vi "Main.vi"() -> ()   [LabVIEW 2013]
doc: "This is the main VI and the GUI for configuring and using the AFM."
uses:
  subvi/simulator/Global Variables.vi
panel:
  out "Function generator waveform display":cluster{dbl[], "Y":dbl[]}(graph)
  out "Sample Size":cluster{"Width (µm)":dbl, "Height (µm)":dbl}={"Width (µm)"=40.0, "Height (µm)"=40.0}
  in  "update X/Y?":bool
  in  "Open simulator?":bool
  out "Rendered Image":T1(plugin-control)
  in  "Settings":T2(tab)=enum."Inkscape Design and Background Image"
  in  "Function generator":T3(array[cluster])=[{"Max Voltage"=10.0, "Min Voltage"=-2.0, "signal type"=enum."Square Wave", "square wave duty cycle (%)"=90.0, "Cycle number"=100.0, "Phase"=0.0}] {"square wave duty cycle (%)" format="%0.2f"}
  in  "Same setting":bool=TRUE
  in  "Same setting":bool=TRUE
  in  "Rectangle Properties":T4(array[cluster])=[{"Speed (um/s)"=2.0, "Direction (For Stroked)"=0, "Start Point"=enum."Bottom Left Corner", "Fill in spacing (um)"=0.3, "Orientation (For Filled)"=enum."Vertical", "Voltage"=5.0}, {"Speed (um/s)"=2.0, "Direction (For Stroked)"=0, "Start Point"=enum."Bottom Left Corner", "Fill in spacing (um)"=0.3, "Orientation (For Filled)"=enum."Vertical", "Voltage"=5.0}, {"Speed (um/s)"=2.0, "Direction (For Stroked)"=0, "Start Point"=enum."Bottom Left Corner", "Fill in spacing (um)"=0.3, "Orientation (For Filled)"=enum."Vertical", "Voltage"=5.0}, {"Speed (um/s)"=2.0, "Direction (For Stroked)"=0, "Start Point"=enum."Bottom Left Corner", "Fill in spacing (um)"=0.3, "Orientation (For Filled)"=enum."Vertical", "Voltage"=5.0}, {"Speed (um/s)"=2.0, "Direction (For Stroked)"=0, "Start Point"=enum."Bottom Left Corner", "Fill in spacing (um)"=0.3, "Orientation (For Filled)"=enum."Vertical", "Voltage"=5.0}, {"Speed (um/s)"=2.0, "Direction (For Stroked)"=0, "Start Point"=enum."Bottom Left Corner", "Fill in spacing (um)"=0.3, "Orientation (For Filled)"=enum."Vertical", "Voltage"=5.0}, {"Speed (um/s)"=2.0, "Direction (For Stroked)"=0, "Start Point"=enum."Bottom Left Corner", "Fill in spacing (um)"=0.3, "Orientation (For Filled)"=enum."Vertical", "Voltage"=5.0}, {"Speed (um/s)"=2.0, "Direction (For Stroked)"=0, "Start Point"=enum."Bottom Left Corner", "Fill in spacing (um)"=0.3, "Orientation (For Filled)"=enum."Vertical", "Voltage"=5.0}, {"Speed (um/s)"=2.0, "Direction (For Stroked)"=0, "Start Point"=enum."Bottom Left Corner", "Fill in spacing (um)"=0.3, "Orientation (For Filled)"=enum."Vertical", "Voltage"=5.0}, {"Speed (um/s)"=2.0, "Direction (For Stroked)"=0, "Start Point"=enum."Bottom Left Corner", "Fill in spacing (um)"=0.3, "Orientation (For Filled)"=enum."Vertical", "Voltage"=5.0}, {"Speed (um/s)"=2.0, "Direction (For Stroked)"=0, "Start Point"=enum."Bottom Left Corner", "Fill in spacing (um)"=0.3, "Orientation (For Filled)"=enum."Vertical", "Voltage"=5.0}, {"Speed (um/s)"=2.0, "Direction (For Stroked)"=0, "Start Point"=enum."Bottom Left Corner", "Fill in spacing (um)"=0.3, "Orientation (For Filled)"=enum."Vertical", "Voltage"=5.0}, {"Speed (um/s)"=2.0, "Direction (For Stroked)"=0, "Start Point"=enum."Bottom Left Corner", "Fill in spacing (um)"=0.3, "Orientation (For Filled)"=enum."Vertical", "Voltage"=5.0}, {"Speed (um/s)"=2.0, "Direction (For Stroked)"=0, "Start Point"=enum."Bottom Left Corner", "Fill in spacing (um)"=0.3, "Orientation (For Filled)"=enum."Vertical", "Voltage"=5.0}, {"Speed (um/s)"=2.0, "Direction (For Stroked)"=0, "Start Point"=enum."Bottom Left Corner", "Fill in spacing (um)"=0.3, "Orientation (For Filled)"=enum."Vertical", "Voltage"=5.0}, {"Speed (um/s)"=2.0, "Direction (For Stroked)"=0, "Start Point"=enum."Bottom Left Corner", "Fill in spacing (um)"=0.3, "Orientation (For Filled)"=enum."Vertical", "Voltage"=5.0}, {"Speed (um/s)"=2.0, "Direction (For Stroked)"=0, "Start Point"=enum."Bottom Left Corner", "Fill in spacing (um)"=0.3, "Orientation (For Filled)"=enum."Vertical", "Voltage"=5.0}, {"Speed (um/s)"=2.0, "Direction (For Stroked)"=0, "Start Point"=enum."Bottom Left Corner", "Fill in spacing (um)"=0.3, "Orientation (For Filled)"=enum."Vertical", "Voltage"=5.0}, {"Speed (um/s)"=2.0, "Direction (For Stroked)"=0, "Start Point"=enum."Bottom Left Corner", "Fill in spacing (um)"=0.3, "Orientation (For Filled)"=enum."Vertical", "Voltage"=5.0}, {"Speed (um/s)"=2.0, "Direction (For Stroked)"=0, "Start Point"=enum."Bottom Left Corner", "Fill in spacing (um)"=0.3, "Orientation (For Filled)"=enum."Vertical", "Voltage"=5.0}, {"Speed (um/s)"=2.0, "Direction (For Stroked)"=0, "Start Point"=enum."Bottom Left Corner", "Fill in spacing (um)"=0.3, "Orientation (For Filled)"=enum."Vertical", "Voltage"=5.0}, {"Speed (um/s)"=2.0, "Direction (For Stroked)"=0, "Start Point"=enum."Bottom Left Corner", "Fill in spacing (um)"=0.3, "Orientation (For Filled)"=enum."Vertical", "Voltage"=5.0}, {"Speed (um/s)"=2.0, "Direction (For Stroked)"=0, "Start Point"=enum."Bottom Left Corner", "Fill in spacing (um)"=0.3, "Orientation (For Filled)"=enum."Vertical", "Voltage"=5.0}, {"Speed (um/s)"=2.0, "Direction (For Stroked)"=0, "Start Point"=enum."Bottom Left Corner", "Fill in spacing (um)"=0.3, "Orientation (For Filled)"=enum."Vertical", "Voltage"=5.0}, {"Speed (um/s)"=2.0, "Direction (For Stroked)"=0, "Start Point"=enum."Bottom Left Corner", "Fill in spacing (um)"=0.3, "Orientation (For Filled)"=enum."Vertical", "Voltage"=5.0}, {"Speed (um/s)"=2.0, "Direction (For Stroked)"=0, "Start Point"=enum."Bottom Left Corner", "Fill in spacing (um)"=0.3, "Orientation (For Filled)"=enum."Vertical", "Voltage"=5.0}, {"Speed (um/s)"=2.0, "Direction (For Stroked)"=0, "Start Point"=enum."Bottom Left Corner", "Fill in spacing (um)"=0.3, "Orientation (For Filled)"=enum."Vertical", "Voltage"=5.0}, {"Speed (um/s)"=2.0, "Direction (For Stroked)"=0, "Start Point"=enum."Bottom Left Corner", "Fill in spacing (um)"=0.3, "Orientation (For Filled)"=enum."Vertical", "Voltage"=5.0}, {"Speed (um/s)"=2.0, "Direction (For Stroked)"=0, "Start Point"=enum."Bottom Left Corner", "Fill in spacing (um)"=0.3, "Orientation (For Filled)"=enum."Vertical", "Voltage"=5.0}, {"Speed (um/s)"=2.0, "Direction (For Stroked)"=0, "Start Point"=enum."Bottom Left Corner", "Fill in spacing (um)"=0.3, "Orientation (For Filled)"=enum."Vertical", "Voltage"=5.0}] {"Direction (For Stroked)" items=["Clockwise", "Counterclockwise"]}
  in  "Inkscape File Path":path=path "C:/AFM/sa02525_test2.svg"
  in  "Background Image File Path (Igor or Bitmap)":path=path "C:/AFM/Sample.ibw"
  in  "Page (for Igor)":i32=1
  in  "Funnel Propeties":T5(array[cluster])=[{"Max Speed (um/s)"=2.0, "Direction (For Stroked)"=0, "Orientation (For Filled)"=enum."Vertical", "Curve smooth segments"=20.0, "Bottom Segments"=20.0, "Voltage"=5.0}, {"Max Speed (um/s)"=2.0, "Direction (For Stroked)"=0, "Orientation (For Filled)"=enum."Vertical", "Curve smooth segments"=20.0, "Bottom Segments"=20.0, "Voltage"=5.0}, {"Max Speed (um/s)"=2.0, "Direction (For Stroked)"=0, "Orientation (For Filled)"=enum."Vertical", "Curve smooth segments"=20.0, "Bottom Segments"=20.0, "Voltage"=5.0}, {"Max Speed (um/s)"=2.0, "Direction (For Stroked)"=0, "Orientation (For Filled)"=enum."Vertical", "Curve smooth segments"=20.0, "Bottom Segments"=20.0, "Voltage"=5.0}, {"Max Speed (um/s)"=2.0, "Direction (For Stroked)"=0, "Orientation (For Filled)"=enum."Vertical", "Curve smooth segments"=20.0, "Bottom Segments"=20.0, "Voltage"=5.0}, {"Max Speed (um/s)"=2.0, "Direction (For Stroked)"=0, "Orientation (For Filled)"=enum."Vertical", "Curve smooth segments"=20.0, "Bottom Segments"=20.0, "Voltage"=5.0}, {"Max Speed (um/s)"=2.0, "Direction (For Stroked)"=0, "Orientation (For Filled)"=enum."Vertical", "Curve smooth segments"=20.0, "Bottom Segments"=20.0, "Voltage"=5.0}, {"Max Speed (um/s)"=2.0, "Direction (For Stroked)"=0, "Orientation (For Filled)"=enum."Vertical", "Curve smooth segments"=20.0, "Bottom Segments"=20.0, "Voltage"=5.0}, {"Max Speed (um/s)"=2.0, "Direction (For Stroked)"=0, "Orientation (For Filled)"=enum."Vertical", "Curve smooth segments"=20.0, "Bottom Segments"=20.0, "Voltage"=5.0}, {"Max Speed (um/s)"=2.0, "Direction (For Stroked)"=0, "Orientation (For Filled)"=enum."Vertical", "Curve smooth segments"=20.0, "Bottom Segments"=20.0, "Voltage"=5.0}, {"Max Speed (um/s)"=2.0, "Direction (For Stroked)"=0, "Orientation (For Filled)"=enum."Vertical", "Curve smooth segments"=20.0, "Bottom Segments"=20.0, "Voltage"=5.0}, {"Max Speed (um/s)"=2.0, "Direction (For Stroked)"=0, "Orientation (For Filled)"=enum."Vertical", "Curve smooth segments"=20.0, "Bottom Segments"=20.0, "Voltage"=5.0}, {"Max Speed (um/s)"=2.0, "Direction (For Stroked)"=0, "Orientation (For Filled)"=enum."Vertical", "Curve smooth segments"=20.0, "Bottom Segments"=20.0, "Voltage"=5.0}, {"Max Speed (um/s)"=2.0, "Direction (For Stroked)"=0, "Orientation (For Filled)"=enum."Vertical", "Curve smooth segments"=20.0, "Bottom Segments"=20.0, "Voltage"=5.0}, {"Max Speed (um/s)"=2.0, "Direction (For Stroked)"=0, "Orientation (For Filled)"=enum."Vertical", "Curve smooth segments"=20.0, "Bottom Segments"=20.0, "Voltage"=5.0}, {"Max Speed (um/s)"=2.0, "Direction (For Stroked)"=0, "Orientation (For Filled)"=enum."Vertical", "Curve smooth segments"=20.0, "Bottom Segments"=20.0, "Voltage"=5.0}, {"Max Speed (um/s)"=2.0, "Direction (For Stroked)"=0, "Orientation (For Filled)"=enum."Vertical", "Curve smooth segments"=20.0, "Bottom Segments"=20.0, "Voltage"=5.0}, {"Max Speed (um/s)"=2.0, "Direction (For Stroked)"=0, "Orientation (For Filled)"=enum."Vertical", "Curve smooth segments"=20.0, "Bottom Segments"=20.0, "Voltage"=5.0}, {"Max Speed (um/s)"=2.0, "Direction (For Stroked)"=0, "Orientation (For Filled)"=enum."Vertical", "Curve smooth segments"=20.0, "Bottom Segments"=20.0, "Voltage"=5.0}, {"Max Speed (um/s)"=2.0, "Direction (For Stroked)"=0, "Orientation (For Filled)"=enum."Vertical", "Curve smooth segments"=20.0, "Bottom Segments"=20.0, "Voltage"=5.0}, {"Max Speed (um/s)"=2.0, "Direction (For Stroked)"=0, "Orientation (For Filled)"=enum."Vertical", "Curve smooth segments"=20.0, "Bottom Segments"=20.0, "Voltage"=5.0}, {"Max Speed (um/s)"=2.0, "Direction (For Stroked)"=0, "Orientation (For Filled)"=enum."Vertical", "Curve smooth segments"=20.0, "Bottom Segments"=20.0, "Voltage"=5.0}, {"Max Speed (um/s)"=2.0, "Direction (For Stroked)"=0, "Orientation (For Filled)"=enum."Vertical", "Curve smooth segments"=20.0, "Bottom Segments"=20.0, "Voltage"=5.0}, {"Max Speed (um/s)"=2.0, "Direction (For Stroked)"=0, "Orientation (For Filled)"=enum."Vertical", "Curve smooth segments"=20.0, "Bottom Segments"=20.0, "Voltage"=5.0}, {"Max Speed (um/s)"=2.0, "Direction (For Stroked)"=0, "Orientation (For Filled)"=enum."Vertical", "Curve smooth segments"=20.0, "Bottom Segments"=20.0, "Voltage"=5.0}, {"Max Speed (um/s)"=2.0, "Direction (For Stroked)"=0, "Orientation (For Filled)"=enum."Vertical", "Curve smooth segments"=20.0, "Bottom Segments"=20.0, "Voltage"=5.0}, {"Max Speed (um/s)"=2.0, "Direction (For Stroked)"=0, "Orientation (For Filled)"=enum."Vertical", "Curve smooth segments"=20.0, "Bottom Segments"=20.0, "Voltage"=5.0}, {"Max Speed (um/s)"=2.0, "Direction (For Stroked)"=0, "Orientation (For Filled)"=enum."Vertical", "Curve smooth segments"=20.0, "Bottom Segments"=20.0, "Voltage"=5.0}, {"Max Speed (um/s)"=2.0, "Direction (For Stroked)"=0, "Orientation (For Filled)"=enum."Vertical", "Curve smooth segments"=20.0, "Bottom Segments"=20.0, "Voltage"=5.0}, {"Max Speed (um/s)"=2.0, "Direction (For Stroked)"=0, "Orientation (For Filled)"=enum."Vertical", "Curve smooth segments"=20.0, "Bottom Segments"=20.0, "Voltage"=5.0}] {"Direction (For Stroked)" items=["Forward", "Backward"]}
  in  "Amplifier Setting":dbl=-15.0
  in  "Path Properties":T6(array[cluster])=[{"Speed (um/s)"=0.4, "Direction"=0, "Orientation (For Filled)"=enum."Vertical", "Curve smooth Segments"=30.0, "Fill in spacing (um)"=0.3, "Start and End voltage"=[{"Numeric"=10.0, "Numeric 2"=10.0}], "Same Voltage"=TRUE, "Function Genrator?"=FALSE}, {"Speed (um/s)"=0.4, "Direction"=0, "Orientation (For Filled)"=enum."Vertical", "Curve smooth Segments"=30.0, "Fill in spacing (um)"=0.3, "Start and End voltage"=[{"Numeric"=10.0, "Numeric 2"=10.0}], "Same Voltage"=TRUE, "Function Genrator?"=FALSE}, {"Speed (um/s)"=0.4, "Direction"=0, "Orientation (For Filled)"=enum."Vertical", "Curve smooth Segments"=30.0, "Fill in spacing (um)"=0.3, "Start and End voltage"=[{"Numeric"=10.0, "Numeric 2"=10.0}], "Same Voltage"=TRUE, "Function Genrator?"=FALSE}, {"Speed (um/s)"=0.4, "Direction"=0, "Orientation (For Filled)"=enum."Vertical", "Curve smooth Segments"=30.0, "Fill in spacing (um)"=0.3, "Start and End voltage"=[{"Numeric"=10.0, "Numeric 2"=10.0}], "Same Voltage"=TRUE, "Function Genrator?"=FALSE}, {"Speed (um/s)"=0.4, "Direction"=0, "Orientation (For Filled)"=enum."Vertical", "Curve smooth Segments"=30.0, "Fill in spacing (um)"=0.3, "Start and End voltage"=[{"Numeric"=10.0, "Numeric 2"=10.0}], "Same Voltage"=TRUE, "Function Genrator?"=FALSE}, {"Speed (um/s)"=0.4, "Direction"=0, "Orientation (For Filled)"=enum."Vertical", "Curve smooth Segments"=30.0, "Fill in spacing (um)"=0.3, "Start and End voltage"=[{"Numeric"=10.0, "Numeric 2"=10.0}], "Same Voltage"=TRUE, "Function Genrator?"=FALSE}, {"Speed (um/s)"=0.4, "Direction"=0, "Orientation (For Filled)"=enum."Vertical", "Curve smooth Segments"=30.0, "Fill in spacing (um)"=0.3, "Start and End voltage"=[{"Numeric"=10.0, "Numeric 2"=10.0}], "Same Voltage"=TRUE, "Function Genrator?"=FALSE}, {"Speed (um/s)"=0.4, "Direction"=0, "Orientation (For Filled)"=enum."Vertical", "Curve smooth Segments"=30.0, "Fill in spacing (um)"=0.3, "Start and End voltage"=[{"Numeric"=10.0, "Numeric 2"=10.0}], "Same Voltage"=TRUE, "Function Genrator?"=FALSE}, {"Speed (um/s)"=0.4, "Direction"=0, "Orientation (For Filled)"=enum."Vertical", "Curve smooth Segments"=30.0, "Fill in spacing (um)"=0.3, "Start and End voltage"=[{"Numeric"=10.0, "Numeric 2"=10.0}], "Same Voltage"=TRUE, "Function Genrator?"=FALSE}, {"Speed (um/s)"=0.4, "Direction"=0, "Orientation (For Filled)"=enum."Vertical", "Curve smooth Segments"=30.0, "Fill in spacing (um)"=0.3, "Start and End voltage"=[{"Numeric"=10.0, "Numeric 2"=10.0}], "Same Voltage"=TRUE, "Function Genrator?"=FALSE}, {"Speed (um/s)"=0.4, "Direction"=0, "Orientation (For Filled)"=enum."Vertical", "Curve smooth Segments"=30.0, "Fill in spacing (um)"=0.3, "Start and End voltage"=[{"Numeric"=10.0, "Numeric 2"=10.0}], "Same Voltage"=TRUE, "Function Genrator?"=FALSE}, {"Speed (um/s)"=0.4, "Direction"=0, "Orientation (For Filled)"=enum."Vertical", "Curve smooth Segments"=30.0, "Fill in spacing (um)"=0.3, "Start and End voltage"=[{"Numeric"=10.0, "Numeric 2"=10.0}], "Same Voltage"=TRUE, "Function Genrator?"=FALSE}, {"Speed (um/s)"=0.4, "Direction"=0, "Orientation (For Filled)"=enum."Vertical", "Curve smooth Segments"=30.0, "Fill in spacing (um)"=0.3, "Start and End voltage"=[{"Numeric"=10.0, "Numeric 2"=10.0}], "Same Voltage"=TRUE, "Function Genrator?"=FALSE}, {"Speed (um/s)"=0.4, "Direction"=0, "Orientation (For Filled)"=enum."Vertical", "Curve smooth Segments"=30.0, "Fill in spacing (um)"=0.3, "Start and End voltage"=[{"Numeric"=10.0, "Numeric 2"=10.0}], "Same Voltage"=TRUE, "Function Genrator?"=FALSE}, {"Speed (um/s)"=0.4, "Direction"=0, "Orientation (For Filled)"=enum."Vertical", "Curve smooth Segments"=30.0, "Fill in spacing (um)"=0.3, "Start and End voltage"=[{"Numeric"=10.0, "Numeric 2"=10.0}], "Same Voltage"=TRUE, "Function Genrator?"=FALSE}, {"Speed (um/s)"=0.4, "Direction"=0, "Orientation (For Filled)"=enum."Vertical", "Curve smooth Segments"=30.0, "Fill in spacing (um)"=0.3, "Start and End voltage"=[{"Numeric"=10.0, "Numeric 2"=10.0}], "Same Voltage"=TRUE, "Function Genrator?"=FALSE}, {"Speed (um/s)"=0.4, "Direction"=0, "Orientation (For Filled)"=enum."Vertical", "Curve smooth Segments"=30.0, "Fill in spacing (um)"=0.3, "Start and End voltage"=[{"Numeric"=10.0, "Numeric 2"=10.0}], "Same Voltage"=TRUE, "Function Genrator?"=FALSE}, {"Speed (um/s)"=0.4, "Direction"=0, "Orientation (For Filled)"=enum."Vertical", "Curve smooth Segments"=30.0, "Fill in spacing (um)"=0.3, "Start and End voltage"=[{"Numeric"=10.0, "Numeric 2"=10.0}], "Same Voltage"=TRUE, "Function Genrator?"=FALSE}, {"Speed (um/s)"=0.4, "Direction"=0, "Orientation (For Filled)"=enum."Vertical", "Curve smooth Segments"=30.0, "Fill in spacing (um)"=0.3, "Start and End voltage"=[{"Numeric"=10.0, "Numeric 2"=10.0}], "Same Voltage"=TRUE, "Function Genrator?"=FALSE}, {"Speed (um/s)"=0.4, "Direction"=0, "Orientation (For Filled)"=enum."Vertical", "Curve smooth Segments"=30.0, "Fill in spacing (um)"=0.3, "Start and End voltage"=[{"Numeric"=10.0, "Numeric 2"=10.0}], "Same Voltage"=TRUE, "Function Genrator?"=FALSE}, {"Speed (um/s)"=0.4, "Direction"=0, "Orientation (For Filled)"=enum."Vertical", "Curve smooth Segments"=30.0, "Fill in spacing (um)"=0.3, "Start and End voltage"=[{"Numeric"=10.0, "Numeric 2"=10.0}], "Same Voltage"=TRUE, "Function Genrator?"=FALSE}, {"Speed (um/s)"=0.4, "Direction"=0, "Orientation (For Filled)"=enum."Vertical", "Curve smooth Segments"=30.0, "Fill in spacing (um)"=0.3, "Start and End voltage"=[{"Numeric"=10.0, "Numeric 2"=10.0}], "Same Voltage"=TRUE, "Function Genrator?"=FALSE}, {"Speed (um/s)"=0.4, "Direction"=0, "Orientation (For Filled)"=enum."Vertical", "Curve smooth Segments"=30.0, "Fill in spacing (um)"=0.3, "Start and End voltage"=[{"Numeric"=10.0, "Numeric 2"=10.0}], "Same Voltage"=TRUE, "Function Genrator?"=FALSE}, {"Speed (um/s)"=0.4, "Direction"=0, "Orientation (For Filled)"=enum."Vertical", "Curve smooth Segments"=30.0, "Fill in spacing (um)"=0.3, "Start and End voltage"=[{"Numeric"=10.0, "Numeric 2"=10.0}], "Same Voltage"=TRUE, "Function Genrator?"=FALSE}, {"Speed (um/s)"=0.4, "Direction"=0, "Orientation (For Filled)"=enum."Vertical", "Curve smooth Segments"=30.0, "Fill in spacing (um)"=0.3, "Start and End voltage"=[{"Numeric"=10.0, "Numeric 2"=10.0}], "Same Voltage"=TRUE, "Function Genrator?"=FALSE}, {"Speed (um/s)"=0.4, "Direction"=0, "Orientation (For Filled)"=enum."Vertical", "Curve smooth Segments"=30.0, "Fill in spacing (um)"=0.3, "Start and End voltage"=[{"Numeric"=10.0, "Numeric 2"=10.0}], "Same Voltage"=TRUE, "Function Genrator?"=FALSE}, {"Speed (um/s)"=0.4, "Direction"=0, "Orientation (For Filled)"=enum."Vertical", "Curve smooth Segments"=30.0, "Fill in spacing (um)"=0.3, "Start and End voltage"=[{"Numeric"=10.0, "Numeric 2"=10.0}], "Same Voltage"=TRUE, "Function Genrator?"=FALSE}, {"Speed (um/s)"=0.4, "Direction"=0, "Orientation (For Filled)"=enum."Vertical", "Curve smooth Segments"=30.0, "Fill in spacing (um)"=0.3, "Start and End voltage"=[{"Numeric"=10.0, "Numeric 2"=10.0}], "Same Voltage"=TRUE, "Function Genrator?"=FALSE}, {"Speed (um/s)"=0.4, "Direction"=0, "Orientation (For Filled)"=enum."Vertical", "Curve smooth Segments"=30.0, "Fill in spacing (um)"=0.3, "Start and End voltage"=[{"Numeric"=10.0, "Numeric 2"=10.0}], "Same Voltage"=TRUE, "Function Genrator?"=FALSE}, {"Speed (um/s)"=0.4, "Direction"=0, "Orientation (For Filled)"=enum."Vertical", "Curve smooth Segments"=30.0, "Fill in spacing (um)"=0.3, "Start and End voltage"=[{"Numeric"=10.0, "Numeric 2"=10.0}], "Same Voltage"=TRUE, "Function Genrator?"=FALSE}] {"Direction" items=["Forward", "Backward"]}
  in  "Same setting":bool=TRUE
  in  "Unselect ALL":bool
  in  "Reset":bool
  in  "Select ALL":bool
  in  "Order":T7(array[cluster])=[{"String"="p0", "Boolean"=TRUE, "Start Voltage"=10.0, "Speed"=4.0000000000000003e-07}, {"String"="p1", "Boolean"=FALSE, "Start Voltage"=10.0, "Speed"=4.0000000000000003e-07}, {"String"="f0", "Boolean"=FALSE, "Start Voltage"=5.0, "Speed"=2e-06}, {"String"="p2", "Boolean"=FALSE, "Start Voltage"=10.0, "Speed"=4.0000000000000003e-07}, {"String"="p3", "Boolean"=FALSE, "Start Voltage"=10.0, "Speed"=4.0000000000000003e-07}] {"Speed" format="%#_6pm/s"}
  in  "Distance Between\n Interpolated Points (um)":dbl=0.005
  in  "Line Width for Simulator (nm)":dbl=0.1
  in  "Display the Wave":bool
  in  "Z Set Point":dbl
  in  "PID close":bool
  out "Offset":T8={"X Offset (µm)"=-1.2812, "Y Offset (µm)"=5.2969}
  in  "Move Z SetPoint":dbl=-1.0
  in  "Withdraw Tip\nwhen finish?":bool=TRUE
  out "Estimated Time\nRequired for Lithography":timestamp=timestamp(-68328.91625119068 s since 1904-01-01) format="%<%H:%M:%S>T"
  in  "Crop?":bool
  in  "Crop Data":T9
  in  "Rotation Angle (degrees CCW)":dbl
  in  "Image Resolution":i32=512
  in  "Inkscape Scaling":T10={"X Scaling (%)"=100.0, "Y Scaling (%)"=100.0}
  in  "Rotation(degree)":dbl
  out "Canvas Size":cluster{"Width":dbl, "Height":dbl}={"Width"=35.0, "Height"=35.0}
  in  "Inkscape Offset":cluster{"X Offset":dbl, "Y Offset":dbl}
  in  "Array":T11(array[cluster])
  out "Lithography Data Out":T12(array[cluster])
  in  "AFM Type":u16(ring)=1 items=["Simulator", "Cypher"]
  in  "Mode":u16(ring) items=["Configure", "Experiment"]
  # "How to use:\n\nFirst you must create a compliant Inkscape sketch with the structures you want to write. The current version can draw funnels, general paths (straight lines or curves), rectangles and general shapes. Next, you should set the correct path in the 'Inkscape Design and Background Image' tab. Next, load an image to use as the background for the simulator and the rendered image. Now change the mode to configure and run (remember to ). The rendered image should show up on the screen and a default order should appear. Change the order to match your needs. In the other tabs, you can adjust various settings for the final outcome. Underneath this settings tab control is the estimated time required for the lithography. When you are ready to run the experiment, select the type of AFM that you are going to be using and specify whether you wish to run the simulator during the experiment. Then change the mode to experiment and hit run."
  # "Speed"
  # "Voltage"
  # "Image is first cropped, then rotated."
  # "Image is first automatically scaled based on the Inkscape window size down to AFM sample size, then scaled \nusing the above controls, then offset."
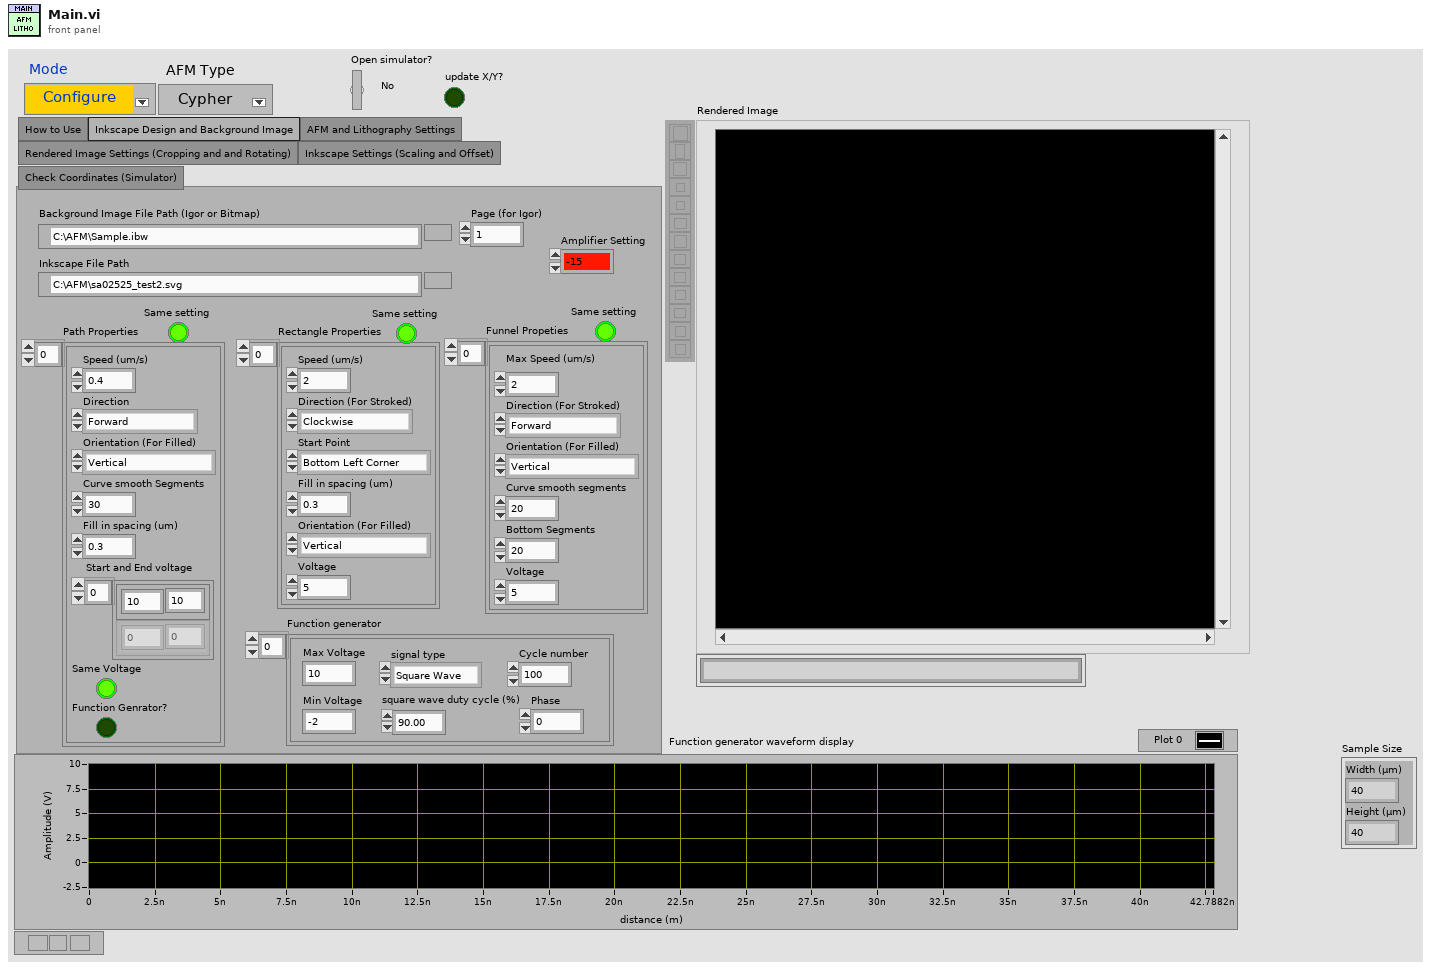
[diagram p1: front panel]
types:
  T1 = typedef "IMAQ Image.ctl" = refnum<image>
  T2 = enum32{"How to Use", "Inkscape Design and Background Image", "AFM and Lithography Settings", "Rendered Image Settings (Cropping and and Rotating)", "Inkscape Settings (Scaling and Offset)", "Check Coordinates (Simulator)"}
  T3 = cluster{"Max Voltage":dbl, "Min Voltage":dbl, "signal type":enum16{"Sine Wave", "Triangle Wave", "Square Wave", "Sawtooth Wave"}, "square wave duty cycle (%)":dbl, "Cycle number":dbl, "Phase":dbl}[]
  T4 = cluster{"Speed (um/s)":dbl, "Direction (For Stroked)":u16, "Start Point":enum16{"Bottom Left Corner", "Bottom Right Corner", "Top Left Corner", "Top Right Corner"}, "Fill in spacing (um)":dbl, "Orientation (For Filled)":enum16{"Horizontal", "Vertical"}, "Voltage":dbl}[]
  T5 = cluster{"Max Speed (um/s)":dbl, "Direction (For Stroked)":u16, "Orientation (For Filled)":enum16{"Horizontal", "Vertical"}, "Curve smooth segments":dbl, "Bottom Segments":dbl, "Voltage":dbl}[]
  T6 = cluster{"Speed (um/s)":dbl, "Direction":u16, "Orientation (For Filled)":enum16{"Horizontal", "Vertical"}, "Curve smooth Segments":dbl, "Fill in spacing (um)":dbl, "Start and End voltage":cluster{"Numeric":dbl, "Numeric 2":dbl}[], "Same Voltage":bool, "Function Genrator?":bool}[]
  T7 = cluster{"String":string, "Boolean":bool, "Start Voltage":dbl, "Speed":dbl}[]
  T8 = cluster{"X Offset (µm)":dbl, "Y Offset (µm)":dbl}
  T9 = cluster{"Left":dbl, "Top":dbl, "Right":dbl, "Bottom":dbl}
  T10 = cluster{"X Scaling (%)":dbl, "Y Scaling (%)":dbl}
  T11 = cluster{"Name":string, "Start V":dbl[], "End V":dbl[]}[]
  T12 = cluster{"Coordinate":cluster{"X":dbl, "Y":dbl}, "Speed":dbl, "Voltage":dbl, "index":i32, "Name":string}[][]
  T13 = cluster{"String":string, "Boolean":bool, "Start Voltage":dbl, "Speed":dbl}
  T14 = cluster{"Speed (um/s)":dbl, "Direction":u16, "Orientation (For Filled)":enum16{"Horizontal", "Vertical"}, "Curve smooth Segments":dbl, "Fill in spacing (um)":dbl, "Start and End voltage":cluster{"Numeric":dbl, "Numeric 2":dbl}[], "Same Voltage":bool, "Function Genrator?":bool}
  T15 = cluster{"Max Speed (um/s)":dbl, "Direction (For Stroked)":u16, "Orientation (For Filled)":enum16{"Horizontal", "Vertical"}, "Curve smooth segments":dbl, "Bottom Segments":dbl, "Voltage":dbl}
  T16 = cluster{"Speed (um/s)":dbl, "Direction (For Stroked)":u16, "Start Point":enum16{"Bottom Left Corner", "Bottom Right Corner", "Top Left Corner", "Top Right Corner"}, "Fill in spacing (um)":dbl, "Orientation (For Filled)":enum16{"Horizontal", "Vertical"}, "Voltage":dbl}
  T17 = typedef "NI_Matrix.lvlib/RealMatrix.ctl" = dbl[][]
  T18 = cluster{"Fill Color":string, "Stroke Color":string, "Width":dbl, "Height":dbl, "X":dbl, "Y":dbl, "Transformation Matrix":T17}[]
  T19 = cluster{"XML":string, "XML":string, "Array of Commands":cluster{"Command Type":string, "Coordinates":cluster{"X":dbl, "Y":dbl}[]}[], "Transformation Matrix":T17, "Order":i32}[]
  T20 = cluster{cluster{"X":dbl, "Y":dbl}[], "Max Speed (um/s)":dbl, "Voltage":cluster{"Voltage":dbl, "Voltage":dbl}[], "Name":string, "Order":i32}[]
  T21 = cluster{cluster{"X":dbl, "Y":dbl}[], "Speed (um/s)":dbl, "Voltage":cluster{"Start":dbl, "End":dbl}[], "Name":string, "Order":i32}[]
  T22 = cluster{"Coordinates":cluster{"X":dbl, "Y":dbl}[], "Speed (um/s)":dbl, "Voltage":cluster{"Start":dbl, "End":dbl}[], "Name":string, "Order":i32}[]
  T23 = cluster{"Name":string, bool, "Start Voltage":dbl, "Start Voltage":dbl}
  T24 = cluster{"Coordinates":cluster{"X":dbl, "Y":dbl}[], "Speed (um/s)":dbl, "Voltage":cluster{"Start":dbl, "End":dbl}[], "Name":string, "Order":i32}
  T25 = cluster{"Point cordinate":cluster{"X":dbl, "Y":dbl}, "Speed":dbl, "Voltage":dbl, "RGB Value":i32, "Name":string}[]
  T26 = cluster{"Coordinate":cluster{"X":dbl, "Y":dbl}, "Speed":dbl, "Voltage":dbl, "RGB Value":i32, "Name":string}[][]
  T27 = cluster{"Coordinate":cluster{"X":dbl, "Y":dbl}, "Speed":dbl, "Voltage":dbl, "RGB Value":i32, "Name":string}
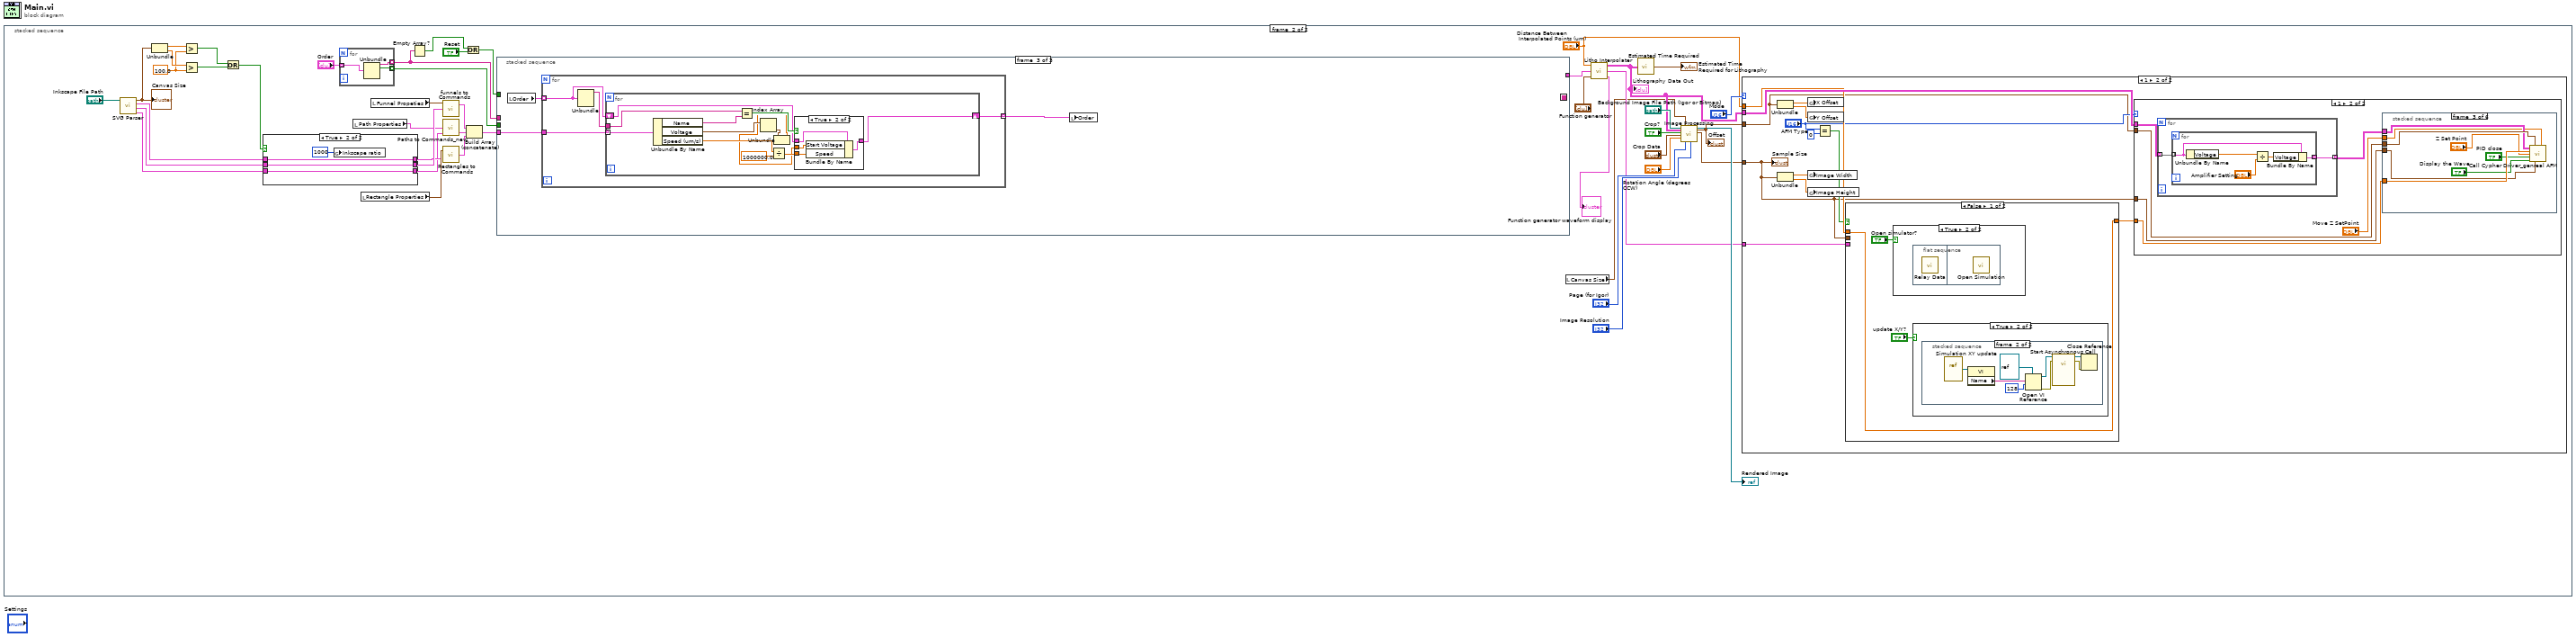
[diagram p0: block diagram]
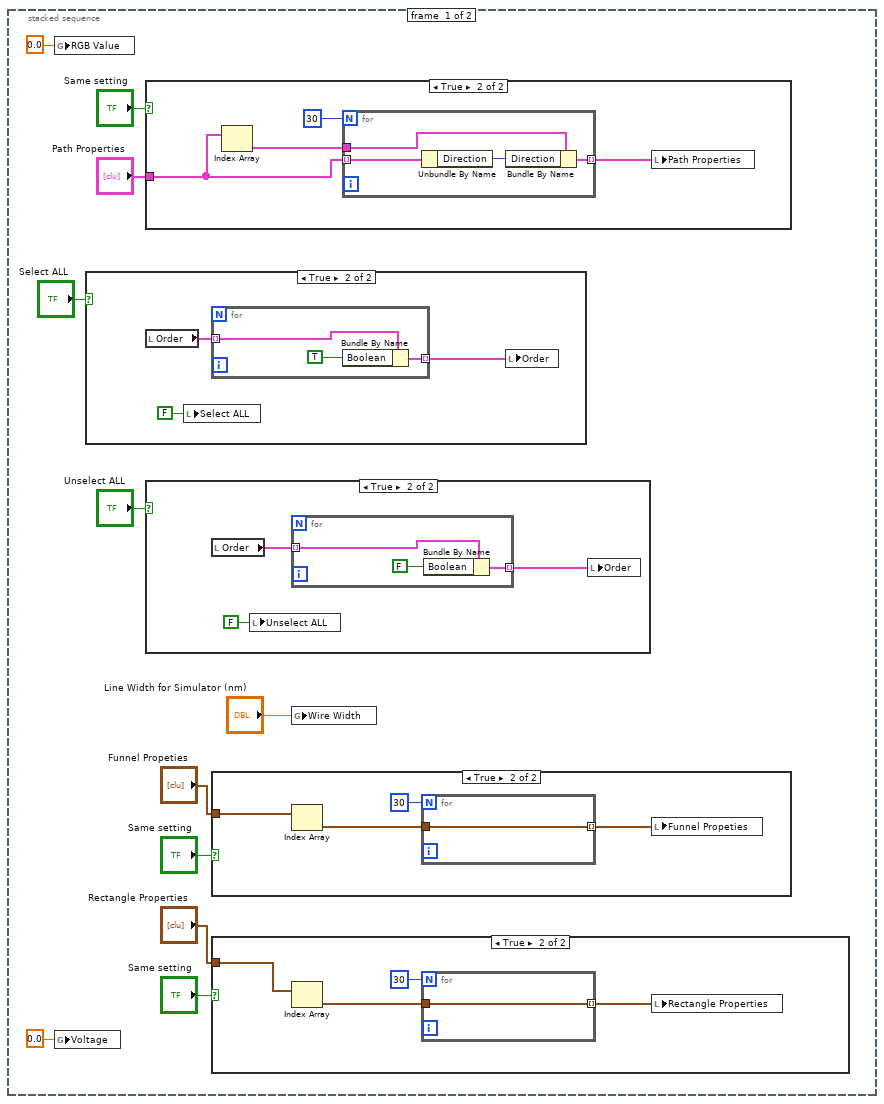
[diagram p2: hidden frame]
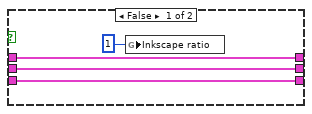
[diagram p8: hidden frame]
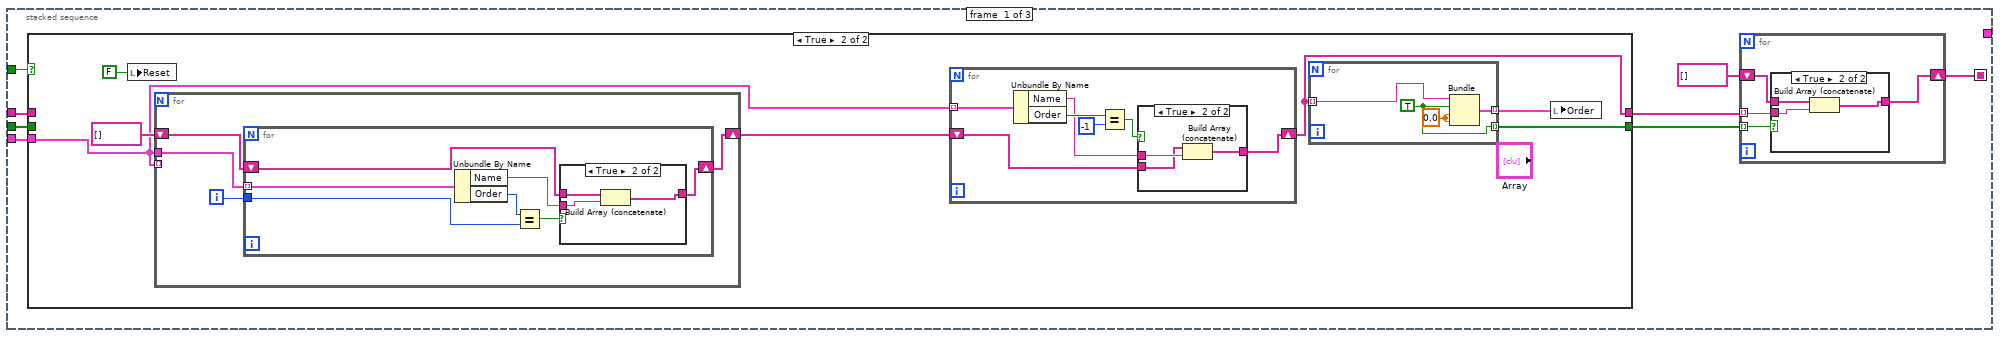
[diagram p9: hidden frame]
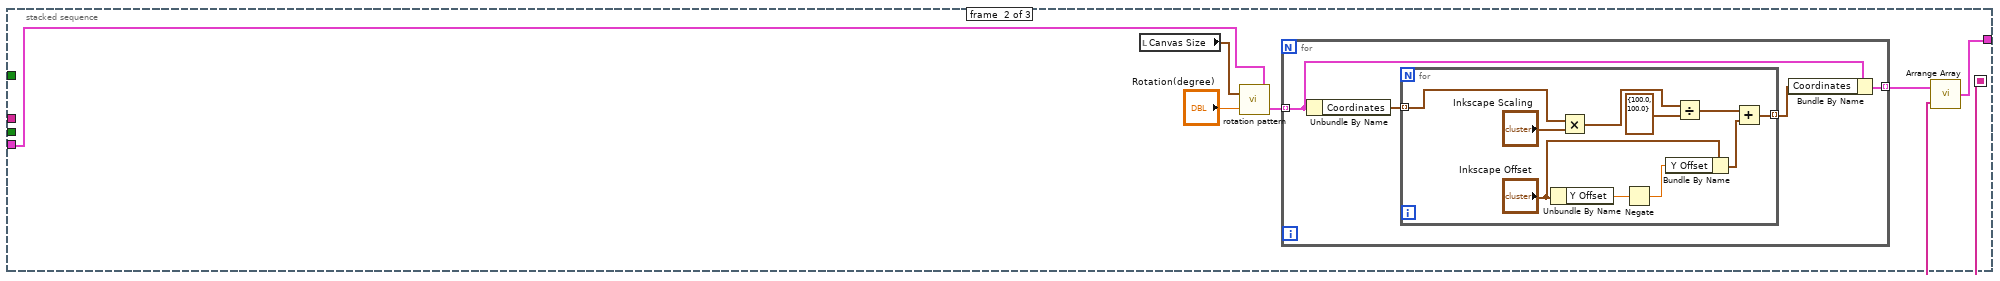
[diagram p14: hidden frame]
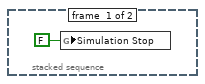
[diagram p18: hidden frame]
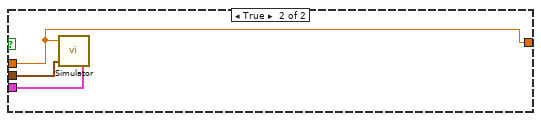
[diagram p20: hidden frame]
diagram:
  n1 = stacked-sequence {
    frame #0 {
      n2 = global write "Global Variables.vi" "RGB Value"(0.0 ("X")) -> ()
      n3 = global write "Global Variables.vi" "Voltage"(0.0 ("X")) -> ()
      n4 = case shown="True" "Select ALL" {
        frame False {
        }
        frame True {
          n5 = local read "Order"() -> (w20:T7)
          n6 = local write "Select ALL"(FALSE ("Select ALL")) -> ()
          n7 = for {
            tunnel: w20 -> [w23] mode=indexing
            tunnel: [w21] -> w19 mode=indexing
            n8 = Bundle By Name(cluster=w23, "Boolean"=TRUE) -> (w21:T13)
          }
          n9 = local write "Order"(w19) -> ()
        }
      }
      n10 = case shown="True" "Same setting" {
        tunnel: "Path Properties" -> [_ w25]
        frame False {
        }
        frame True {
          n11 = Index Array(array=w25) -> (element=w24:T14)  [unwired: 1 in]
          n12 = for {
            N: 30 -> [_]
            tunnel: w25 -> [w31] mode=indexing
            tunnel: [w28] -> w26 mode=indexing
            tunnel: w24 -> [w30]
            n13 = Unbundle By Name(w31) -> ("Direction"=w29:u16)
            n14 = Bundle By Name(cluster=w30, "Direction"=w29) -> (w28:T14)
          }
          n15 = local write "Path Properties"(w26) -> ()
        }
      }
      n16 = case shown="True" "Unselect ALL" {
        frame False {
        }
        frame True {
          n17 = local read "Order"() -> (w14:T7)
          n18 = local write "Unselect ALL"(FALSE ("Select ALL")) -> ()
          n19 = for {
            tunnel: w14 -> [w17] mode=indexing
            tunnel: [w15] -> w13 mode=indexing
            n20 = Bundle By Name(cluster=w17, "Boolean"=FALSE) -> (w15:T13)
          }
          n21 = local write "Order"(w13) -> ()
        }
      }
      n22 = case shown="True" "Same setting" {
        tunnel: "Funnel Propeties" -> [_ w35]
        frame False {
        }
        frame True {
          n23 = Index Array(array=w35) -> (element=w34:T15)  [unwired: 1 in]
          n24 = for {
            N: 30 -> [_]
            tunnel: w34 -> [w36]
            tunnel: [w36] -> w32 mode=indexing
          }
          n25 = local write "Funnel Propeties"(w32) -> ()
        }
      }
      n26 = case shown="True" "Same setting" {
        tunnel: "Rectangle Properties" -> [_ w40]
        frame False {
        }
        frame True {
          n27 = Index Array(array=w40) -> (element=w39:T16)  [unwired: 1 in]
          n28 = for {
            N: 30 -> [_]
            tunnel: w39 -> [w41]
            tunnel: [w41] -> w37 mode=indexing
          }
          n29 = local write "Rectangle Properties"(w37) -> ()
        }
      }
      n30 = global write "Global Variables.vi" "Wire Width"("Line Width for Simulator (nm)") -> ()
    }
    frame #1 {
      w55 = 100.0 ("y")
      n31 = call "SVG Parser.vi"("XML File Path"="Inkscape File Path") -> ("Image Size"=w58:cluster{"Width":dbl, "Height":dbl}, "rects"=w49:T18, "Funnel"=w51:T19, "Path"=w50:T19)  [unwired: 2 in, 1 out]
      "Canvas Size" <- w58
      n32 = Unbundle(w58) -> ("Width"=w57:dbl, "Height"=w56:dbl)
      n33 = Greater?(x=w57, y=w55) -> (0:w54:bool)
      n34 = Greater?(x=w56, y=w55) -> (0:w53:bool)
      n35 = Or(x=w54, y=w53) -> (x .or. y?=w52:bool)
      n36 = case shown="True" w52 {
        tunnel: w49 -> [w88 w94]
        tunnel: w51 -> [w90 w93]
        tunnel: w50 -> [w89 w92]
        tunnel: [w88 w94] -> w47
        tunnel: [w90 w93] -> w48
        tunnel: [w89 w92] -> w46
        frame False {
          n37 = global write "Global Variables.vi" "Inkscape ratio"(1) -> ()
        }
        frame True {
          n38 = global write "Global Variables.vi" "Inkscape ratio"(1000) -> ()
        }
      }
      n39 = for {
        tunnel: "Order" -> [w197] mode=indexing
        tunnel: [w196] -> w72 mode=indexing
        tunnel: [w195] -> w71 mode=indexing
        n40 = Unbundle(w197) -> ("String"=w196:string, "Boolean"=w195:bool)  [unwired: 2 out]
      }
      n41 = local read "Path Properties"() -> (w44:T6)
      n42 = local read "Rectangle Properties"() -> (w62:T4)
      n43 = local read "Funnel Propeties"() -> (w63:T5)
      n44 = Empty Array?(array=w72) -> (empty?=w77:bool)
      n45 = call "funnels to Commands.vi"("Funnel"=w48, "Funnel Propeties"=w63) -> ("Lithography information"=w68:T20)  [unwired: 2 in]
      n46 = call "Paths to Commands_new.vi"("Path"=w46, "Path Properties"=w44) -> ("Lithography information"=w67:T21)  [unwired: 1 in, 1 out]
      n47 = call "Rectangles to Commands.vi"("rects"=w47, "Rectangle Properties"=w62) -> ("Lithography information"=w66:T22)
      n48 = Or(x=w77, y="Reset") -> (x .or. y?=w79:bool)
      n49 = Build Array (concatenate)(w68, w67, w66) -> (w45:T22)
      n50 = stacked-sequence {
        seq-local: [w98 _ _] -> [_ w156 _]
        tunnel: w45 -> [w101 w154 w171]
        tunnel: w79 -> [w102 _ _]
        tunnel: w72 -> [w100 _ _]
        tunnel: w71 -> [w97 _ _]
        tunnel: [_ w155 _] -> w59
        frame #0 {
          n51 = case shown="True" w102 {
            tunnel: w101 -> [_ w115]
            tunnel: [w112 w114] -> w99
            tunnel: w100 -> [w112 _]
            tunnel: w97 -> [w111 _]
            tunnel: [w111 w119] -> w96
            frame False {
            }
            frame True {
              n52 = local write "Reset"(FALSE ("Reset")) -> ()
              n53 = for {
                tunnel: w115 -> [w134]
                shift-right: [w133] -> w116
                shift-left: string[] [] -> [w131]
                tunnel: w115 -> [_] mode=indexing
                i -> [w132]
                n54 = for {
                  tunnel: w134 -> [w141] mode=indexing
                  tunnel: w132 -> [w139]
                  shift-right: [w136] -> w133
                  shift-left: w131 -> [w135]
                  n55 = Unbundle By Name(w141) -> ("Name"=w137:string, "Order"=w140:i32)
                  n56 = Equal?(x=w140, y=w139) -> (x = y?=w138:bool)
                  n57 = case shown="True" w138 {
                    tunnel: w137 -> [_ w145]
                    tunnel: [w142 w144] -> w136
                    tunnel: w135 -> [w142 w143]
                    frame False {
                    }
                    frame True {
                      n58 = Build Array (concatenate)(w143, w145) -> (w144:string[])
                    }
                  }
                }
              }
              n59 = for {
                tunnel: w115 -> [w126] mode=indexing
                shift-right: [w122] -> w114
                shift-left: w116 -> [w121]
                n60 = Unbundle By Name(w126) -> ("Name"=w123:string, "Order"=w125:i32)
                n61 = Equal?(x=w125, y=-1) -> (x = y?=w124:bool)
                n62 = case shown="True" w124 {
                  tunnel: w123 -> [_ w130]
                  tunnel: [w127 w129] -> w122
                  tunnel: w121 -> [w127 w128]
                  frame False {
                  }
                  frame True {
                    n63 = Build Array (concatenate)(w128, w130) -> (w129:string[])
                  }
                }
              }
              n64 = for {
                tunnel: w114 -> [w149] mode=indexing
                tunnel: [w148] -> w119 mode=indexing
                tunnel: [w147] -> w113 mode=indexing
                w146 = 0.0 ("Start Voltage")
                w148 = TRUE
                n65 = Bundle("Name"=w149, w148, "Start Voltage"=w146, "Start Voltage"=w146) -> (w147:T23)  [unwired: 1 in]
              }
              n66 = local write "Order"(w113) -> ()
            }
          }
          n67 = for {
            tunnel: w99 -> [w106] mode=indexing
            tunnel: w96 -> [w103] mode=indexing
            shift-right: [w105] -> w98
            shift-left: string[] [] -> [w104]
            n68 = case shown="True" w103 {
              tunnel: w106 -> [_ w110]
              tunnel: [w107 w109] -> w105
              tunnel: w104 -> [w107 w108]
              frame False {
              }
              frame True {
                n69 = Build Array (concatenate)(w108, w110) -> (w109:string[])
              }
            }
          }
        }
        frame #1 {
          n70 = local read "Canvas Size"() -> (w152:cluster{"Width":dbl, "Height":dbl})
          n71 = call "rotation pattern.vi"("Rotation array"=w154, "Rotation(degree)"="Rotation(degree)", "Inkscape Image Size"=w152) -> ("Rotated array"=w151:T22)
          n72 = for {
            tunnel: w151 -> [w159] mode=indexing
            tunnel: [w157] -> w150 mode=indexing
            n73 = Unbundle By Name(w159) -> ("Coordinates"=w160:cluster{"X":dbl, "Y":dbl}[])
            n74 = for {
              tunnel: [w167] -> w158 mode=indexing
              tunnel: w160 -> [w166] mode=indexing
              n75 = Unbundle By Name("Inkscape Offset") -> ("Y Offset"=w163:dbl)
              n76 = Multiply(x=w166, y="Inkscape Scaling") -> (x*y=w170:cluster{dbl, dbl})
              n77 = Negate(x=w163) -> (-x=w164:dbl)
              n78 = Bundle By Name(cluster="Inkscape Offset", "Y Offset"=w164) -> (w161:cluster{"X Offset":dbl, "Y Offset":dbl})
              n79 = Divide(x=w170, y=cluster{dbl, dbl} {100.0, 100.0}) -> (x/y=w168:cluster{dbl, dbl})
              n80 = Add(x=w168, y=w161) -> (x+y=w167:cluster{dbl, dbl})
            }
            n81 = Bundle By Name(cluster=w159, "Coordinates"=w158) -> (w157:T24)
          }
          n82 = call "Arrange Array.vi"("Order"=w156, "Arrange array"=w150) -> ("Arranged array"=w155:T22)
        }
        frame #2 {
          n83 = local read "Order"() -> (w173:T7)
          n84 = for {
            tunnel: w173 -> [w175] mode=indexing
            tunnel: [w176] -> w172 mode=indexing
            tunnel: w171 -> [w174]
            n85 = Unbundle(w175) -> ("String"=w177:string)  [unwired: 3 out]
            n86 = for {
              tunnel: w177 -> [w188]
              shift-right: [w186] -> w176
              shift-left: w175 -> [w185]
              tunnel: w174 -> [w184] mode=indexing
              n87 = Unbundle By Name(w184) -> ("Name"=w189:string, "Voltage"=w180:cluster{"Start":dbl, "End":dbl}[], "Speed (um/s)"=w183:dbl)
              n88 = Equal?(x=w188, y=w189) -> (x = y?=w187:bool)
              n89 = Index Array(array=w180) -> (element=w179:cluster{"Start":dbl, "End":dbl})  [unwired: 1 in]
              n90 = Divide(x=w183, y=1000000.0) -> (x/y=w181:dbl)
              n91 = Unbundle(w179) -> ("Start"=w178:dbl)  [unwired: 1 out]
              n92 = case shown="True" w187 {
                tunnel: w185 -> [w190 w194]
                tunnel: w178 -> [_ w193]
                tunnel: [w190 w192] -> w186
                tunnel: w181 -> [_ w191]
                frame False {
                }
                frame True {
                  n93 = Bundle By Name(cluster=w194, "Start Voltage"=w193, "Speed"=w191) -> (w192:T13)
                }
              }
            }
          }
          n94 = local write "Order"(w172) -> ()
        }
      }
      n95 = local read "Canvas Size"() -> (w60:cluster{"Width":dbl, "Height":dbl})
      n96 = call "Litho Interpolater.vi"("Function generator"="Function generator", "Lithography Data In"=w59, "Distance"="Distance Between\n Interpolated Points (um)") -> ("XY Graph"=→"Function generator waveform display":cluster{dbl[], "Y":dbl[]}, "Simulator Data Out"=w61:T25, "Lithography Data Out"=w74:T26)
      "Lithography Data Out" <- w74
      n97 = call "Estimated Time Required.vi"("Lithography Information"=w74) -> ("Estimated Time Required"=→"Estimated Time\nRequired for Lithography":timestamp)
      n98 = call "Image Processing.vi"("File Path"="Background Image File Path (Igor or Bitmap)", "Lithography Information"=w74, "Crop?"="Crop?", "Crop Data"="Crop Data", "Angle (degrees)"="Rotation Angle (degrees CCW)", "Size"=w60, "Page"="Page (for Igor)", "Resolution"="Image Resolution") -> ("Image Out"=→"Rendered Image":T1, "Offset"=w64:T8, "Sample Size"=w65:cluster{"Width (µm)":dbl, "Height (µm)":dbl})  [unwired: 8 in, 1 out]
      "Offset" <- w64
      n99 = case shown="1" "Mode" {
        tunnel: w74 -> [_ w210]
        tunnel: "Distance Between\n Interpolated Points (um)" -> [_ w209]
        tunnel: w65 -> [_ w201]
        tunnel: w64 -> [_ w198]
        tunnel: w61 -> [_ w205]
        frame 0, Default {
        }
        frame 1 {
          n100 = Unbundle(w198) -> ("X Offset (µm)"=w200:dbl, "Y Offset (µm)"=w199:dbl)
          n101 = Unbundle(w201) -> ("Width (µm)"=w202:dbl, "Height (µm)"=w203:dbl)
          n102 = global write "Global Variables.vi" "X Offset"(w200) -> ()
          n103 = global write "Global Variables.vi" "Y Offset"(w199) -> ()
          n104 = global write "Global Variables.vi" "Image Width"(w202) -> ()
          n105 = global write "Global Variables.vi" "Image Height"(w203) -> ()
          n106 = Equal?(x="AFM Type", y=u16 0) -> (x = y?=w207:bool)
          n107 = case shown="False" w207 {
            tunnel: w209 -> [w212 w223]
            tunnel: w201 -> [_ w225]
            tunnel: w205 -> [_ w224]
            tunnel: [w212 w223] -> w204
            frame False {
              n108 = case shown="True" "Open simulator?" {
                frame False {
                }
                frame True {
                  n109 = flat-sequence {
                    frame #0 {
                      n110 = call "Relay Data.vi"() -> ()  [unwired: 12 in]
                    }
                    frame #1 {
                      n111 = call "Open Simulation.vi"() -> ()  [unwired: 12 in]
                    }
                  }
                }
              }
              n112 = case shown="True" "update X/Y?" {
                frame False {
                }
                frame True {
                  n113 = stacked-sequence {
                    frame #0 {
                      n114 = global write "Global Variables.vi" "Simulation Stop"(FALSE ("Simulation Stop")) -> ()
                    }
                    frame #1 {
                      n115 = vi-ref "Simulation XY update.vi"() -> (w221:refnum<vi>)
                      n116 = property class="VI"(reference=w221) -> ("Name"=w220:string)  [unwired: 1 in, 2 out]
                      n117 = Open VI Reference(type specifier VI Refnum (for type only)=refnum<vi> refnum, vi path=w220, options=128) -> (vi reference=w218:refnum<vi>, error out=w217:errorcluster)  [unwired: 3 in]
                      n118 = call-by-ref "Start Asynchronous Call"(reference=w218, error in=w217) -> (reference out=w215:refnum<vi>, error out=w216:errorcluster)  [unwired: 12 in]
                      n119 = Close Reference(reference=w215, error in (no error)=w216) -> ()  [unwired: 1 out]
                    }
                  }
                }
              }
            }
            frame True {
              n120 = call "Simulator.vi"("Simulator Data Out"=w224, "Sample Size"=w225, "Distance Between Interpolated Points"=w223) -> ()  [unwired: 2 in, 1 out]
            }
          }
          n121 = case shown="1" "AFM Type" {
            tunnel: w210 -> [_ w230]
            tunnel: w204 -> [_ w231]
            tunnel: w201 -> [_ w228]
            tunnel: w198 -> [_ w227]
            frame 0, Default {
            }
            frame 1 {
              n122 = for {
                tunnel: w230 -> [w257] mode=indexing
                tunnel: [w256] -> w229 mode=indexing
                n123 = for {
                  tunnel: w257 -> [w259] mode=indexing
                  tunnel: [w258] -> w256 mode=indexing
                  n124 = Unbundle By Name(w259) -> ("Voltage"=w262:dbl)
                  n125 = Divide(x=w262, y="Amplifier Setting") -> (x/y=w260:dbl)
                  n126 = Bundle By Name(cluster=w259, "Voltage"=w260) -> (w258:T27)
                }
              }
              n127 = stacked-sequence {
                tunnel: w229 -> [_ _ w238 _ _ _]
                tunnel: w228 -> [_ _ w242 _ _ _]
                tunnel: w231 -> [_ _ w244 _ _ _]
                tunnel: w227 -> [_ _ w243 _ _ _]
                tunnel: "Move Z SetPoint" -> [_ _ w237 _ w247 _]
                frame #0 {
                  n128 = stacked-sequence {
                    frame #0 {
                      n129 = global write "Global Variables.vi" "Read data"(FALSE ("Read data")) -> ()
                    }
                    frame #1 {
                      n130 = Wait (ms)(milliseconds to wait=u32 500) -> ()  [unwired: 1 out]
                    }
                    frame #2 {
                      w235 = u16 0 items=["OutA_52kHz", "OutB_52kHz", "OutC_78Hz", "PiezoX", "PiezoY", "PiezoZ", "DDS_Frequency1", "DDS_Frequency2", "DDS_Amplitude1", "DDS_Amplitude2", "DDS_DCOffset", "\"Setpoint%PIDSLoop.3\"", "\"Setpoint%PIDSLoop.4\"", ""] ("Output")
                      n131 = call "Set value.vi"("Value"=0.0, "Output"=w235) -> ()  [unwired: 9 in, 1 out]
                    }
                    frame #3 {
                      n132 = global write "Global Variables.vi" "Read data"(TRUE ("Read data")) -> ()
                    }
                  }
                }
                frame #1 {
                }
                frame #2 {
                  n133 = call "Call Cypher Driver_genreal AFM.vi"("Output Array"=w238, "Offset"=w243, "Move Z SetPoint"=w237, "Distance Between Interpolated Points (nm)"=w244, "Z Set Point (For Cypher AFM)"="Z Set Point", "PID close"="PID close", "Display the Wave (Cypher AFM)"="Display the Wave", "Image Size"=w242) -> ()  [unwired: 8 in]
                }
                frame #3 {
                  n134 = global write "Global Variables.vi" "Read data"(FALSE ("Read data")) -> ()
                  n135 = Wait (ms)(milliseconds to wait=u32 500) -> ()  [unwired: 1 out]
                }
                frame #4 {
                  n136 = case shown="True" "Withdraw Tip\nwhen finish?" {
                    tunnel: w247 -> [_ w249]
                    frame False {
                    }
                    frame True {
                      n137 = call "Tip touchdown.vi"("Z SetPoint"=w249) -> ()  [unwired: 11 out]
                      n138 = Wait (ms)(milliseconds to wait=u32 500) -> ()  [unwired: 1 out]
                    }
                  }
                }
                frame #5 {
                  n139 = stacked-sequence {
                    frame #0 {
                      n140 = Wait (ms)(milliseconds to wait=u32 2000) -> ()  [unwired: 1 out]
                    }
                    frame #1 {
                      w253 = u16 0 items=["OutA_52kHz", "OutB_52kHz", "OutC_78Hz", "PiezoX", "PiezoY", "PiezoZ", "DDS_Frequency1", "DDS_Frequency2", "DDS_Amplitude1", "DDS_Amplitude2", "DDS_DCOffset", "\"Setpoint%PIDSLoop.3\"", "\"Setpoint%PIDSLoop.4\"", ""] ("Output")
                      n141 = call "Set value.vi"("Value"=0.0, "Output"=w253) -> ()  [unwired: 9 in, 1 out]
                    }
                    frame #2 {
                      n142 = global write "Global Variables.vi" "Read data"(TRUE ("Read data")) -> ()
                      n143 = global write "Global Variables.vi" "Simulation Stop"(TRUE ("Simulation Stop")) -> ()
                    }
                  }
                }
              }
            }
          }
          "Sample Size" <- w201
        }
      }
    }
  }
